vi "image location settings to tracker location settings.vi"(9 "scan settings":T2, 10 "location constraints":T3(array[cluster])) -> (2 "spot location constraints":T1(array[cluster]))   [LabVIEW 2010]
uses:
  scan_specification_tagResonant.ctl
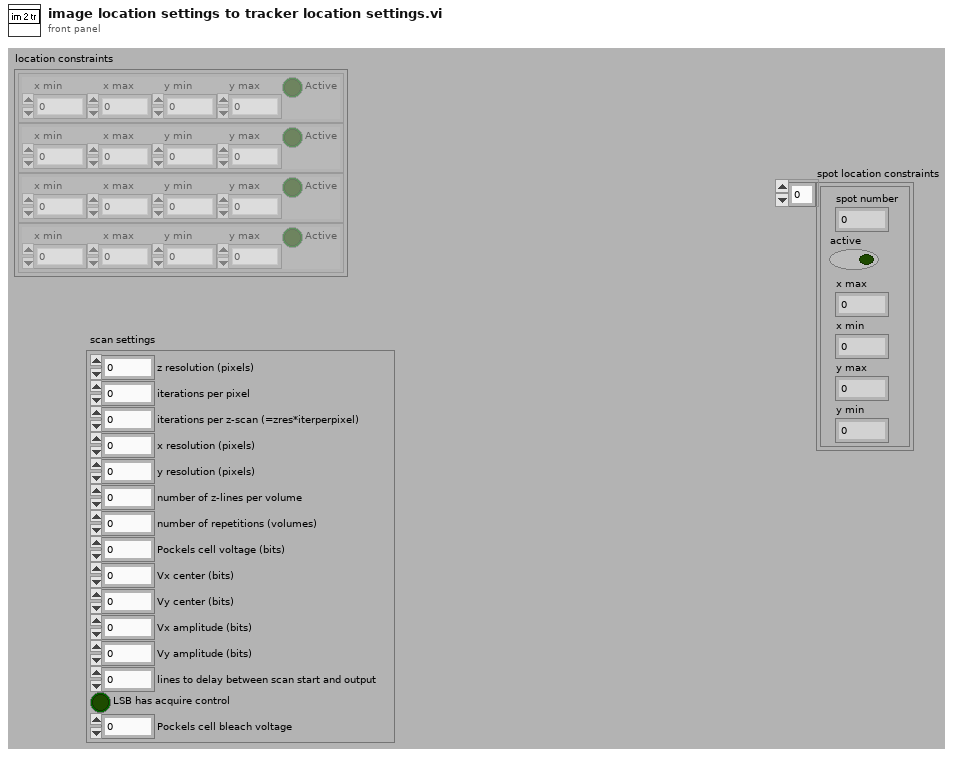
[diagram p1: front panel]
types:
  T1 = cluster{"spot number":i8, "active":bool, "x max":i16, "x min":i16, "y max":i16, "y min":i16}[]
  T2 = typedef "scan_specification_tagResonant.ctl" = cluster{"z resolution (pixels)":u16, "iterations per pixel":u16, "iterations per z-scan (=zres*iterperpixel)":u16, "x resolution (pixels)":u16, "y resolution (pixels)":u16, "number of z-lines per volume":u16, "number of repetitions (volumes)":i32, "Pockels cell voltage (bits)":i16, "Vx center (bits)":i16, "Vy center (bits)":i16, "Vx amplitude (bits)":i16, "Vy amplitude (bits)":i16, "lines to delay between scan start and output":u16, "LSB has acquire control":bool, "Pockels cell bleach voltage":i16}
  T3 = cluster{"x min":i32, "x max":i32, "y min":i32, "y max":i32, "Active":bool}[]
  T4 = cluster{"spot number":i8, "active":bool, "x max":i16, "x min":i16, "y max":i16, "y min":i16}
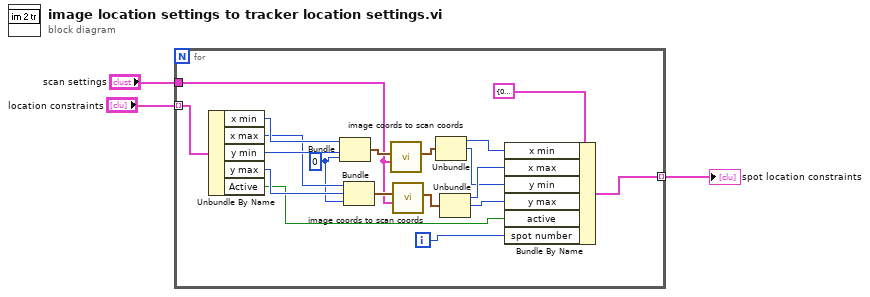
[diagram p0: block diagram]
diagram:
  n1 = for {
    tunnel: "location constraints" -> [w12] mode=indexing
    tunnel: "scan settings" -> [w15]
    tunnel: [w8] -> w1 mode=indexing
    i -> [w5]
    w18 = 0 ("y min")
    n2 = Unbundle By Name(w12) -> ("x min"=w22:i32, "x max"=w20:i32, "y min"=w21:i32, "y max"=w19:i32, "Active"=w6:bool)
    n3 = Bundle("x min"=w22, "y min"=w21, "y min"=w18) -> (w17:cluster{"x min":i32, "y min":i32, "y min":i32})  [unwired: 1 in]
    n4 = Bundle("x max"=w20, "y max"=w19, "y min"=w18) -> (w16:cluster{"x max":i32, "y max":i32, "y min":i32})  [unwired: 1 in]
    n5 = call "image coords to scan coords.vi"("scan settings"=w15, "im location"=w17) -> ("tracking location"=w14:cluster{"x":i16, "y":i16, "z":i16})  [unwired: 9 in]
    n6 = call "image coords to scan coords.vi"("scan settings"=w15, "im location"=w16) -> ("tracking location"=w13:cluster{"x":i16, "y":i16, "z":i16})  [unwired: 9 in]
    n7 = Unbundle(w14) -> ("x"=w11:i16, "y"=w9:i16)  [unwired: 1 out]
    n8 = Unbundle(w13) -> ("x"=w10:i16, "y"=w4:i16)  [unwired: 1 out]
    n9 = Bundle By Name(cluster=T4 {"spot number"=0, "active"=FALSE, "x max"=0, "x min"=0, "y max"=0, "y min"=0} ("spot location constraint"), "x min"=w11, "x max"=w10, "y min"=w9, "y max"=w4, "active"=w6, "spot number"=w5) -> (w8:T4)
  }
  "spot location constraints" <- w1
